vi "SubVI_Assignment3.vi"() -> ()   [LabVIEW 2022 SP3]
panel:
  in  "Ring":u16(ring) items=["square", "triangle", "sinusoidal"]
  in  "stop":bool
  out "Waveform Chart":dbl(graph)
  in  "Amplitude":dbl
  in  "Signal Freq":dbl
  in  "Sampling Time Interval (s)":dbl
  # "Lab 1: Assignment 3"
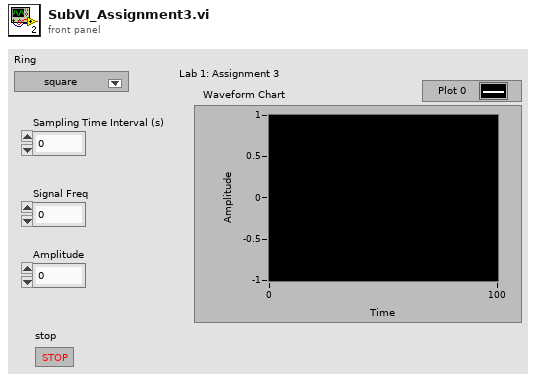
[diagram p1: front panel]
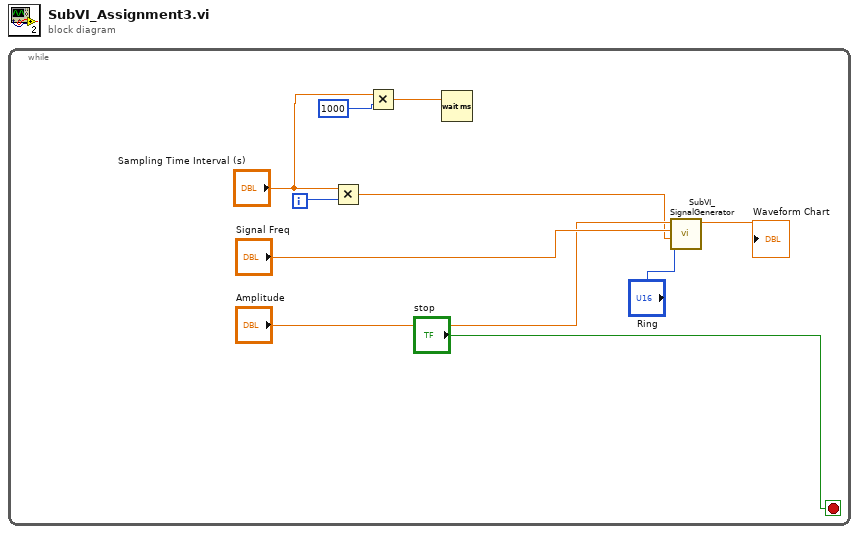
[diagram p0: block diagram]
diagram:
  n1 = while {
    i -> [w5]
    stop <- "stop" stop-if-true
    n2 = Multiply(x="Sampling Time Interval (s)", y=w5) -> (x*y=w2:dbl)
    n3 = Multiply(x="Sampling Time Interval (s)", y=1000) -> (x*y=w3:dbl)
    n4 = Wait (ms)(milliseconds to wait=w3) -> ()  [unwired: 1 out]
    n5 = call "SubVI_SignalGenerator.vi"("Signal Type"="Ring", "Time"=w2, "Freq"="Signal Freq", "Amplitude"="Amplitude") -> ("Signal Gen"=→"Waveform Chart":dbl)  [unwired: 7 in]
  }
